vi "fill channelselector from array.vi"(1 "channel  names":string[](array[string])) -> (0 "channel selector string and values":cluster{"String":string, "Value":u16}[](array[cluster]))   [LabVIEW 2015]
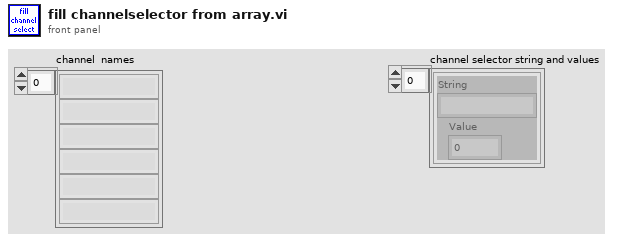
[diagram p1: front panel]
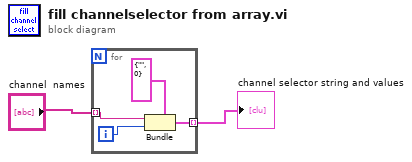
[diagram p0: block diagram]
diagram:
  n1 = for {
    tunnel: "channel  names" -> [w6] mode=indexing
    tunnel: [w4] -> w1 mode=indexing
    i -> [w5]
    n2 = Bundle(cluster=cluster{"String":string, "Value":u16} {"String"="", "Value"=0} ("Cluster"), "String"=w6, "Value"=w5) -> (w4:cluster{"String":string, "Value":u16})
  }
  "channel selector string and values" <- w1
